vi "S8300E_BP_SoftRest_WIH.vi"() -> ()   [LabVIEW 2011]
panel:
  out "Prelog1":string
  out "prelog2":string
  out "log2":string
  out "FinalLog1":string
  out "LOG1":string
  out "FinalLog2":string
  out "Test CMD":T1(array[cluster])
  out "Init CMD":T2(array[cluster])
  out "VISA Handle Array":refnum<visa-resource-name>[](array[refnum])
  out "VISA6":refnum<visa-resource-name>
  out "VISA9":refnum<visa-resource-name>
  out "BEGIN TIME":u32
  out "進行狀況":string
  # "Error Code:BP-RST"
  # "S8300E BackPlane  SW Reset"
  # "2015-5-28"
  # "PC Com9 Baud  115200 -->S8300E MB\nPC COM6 Baud 115200 -->Test Board UART"
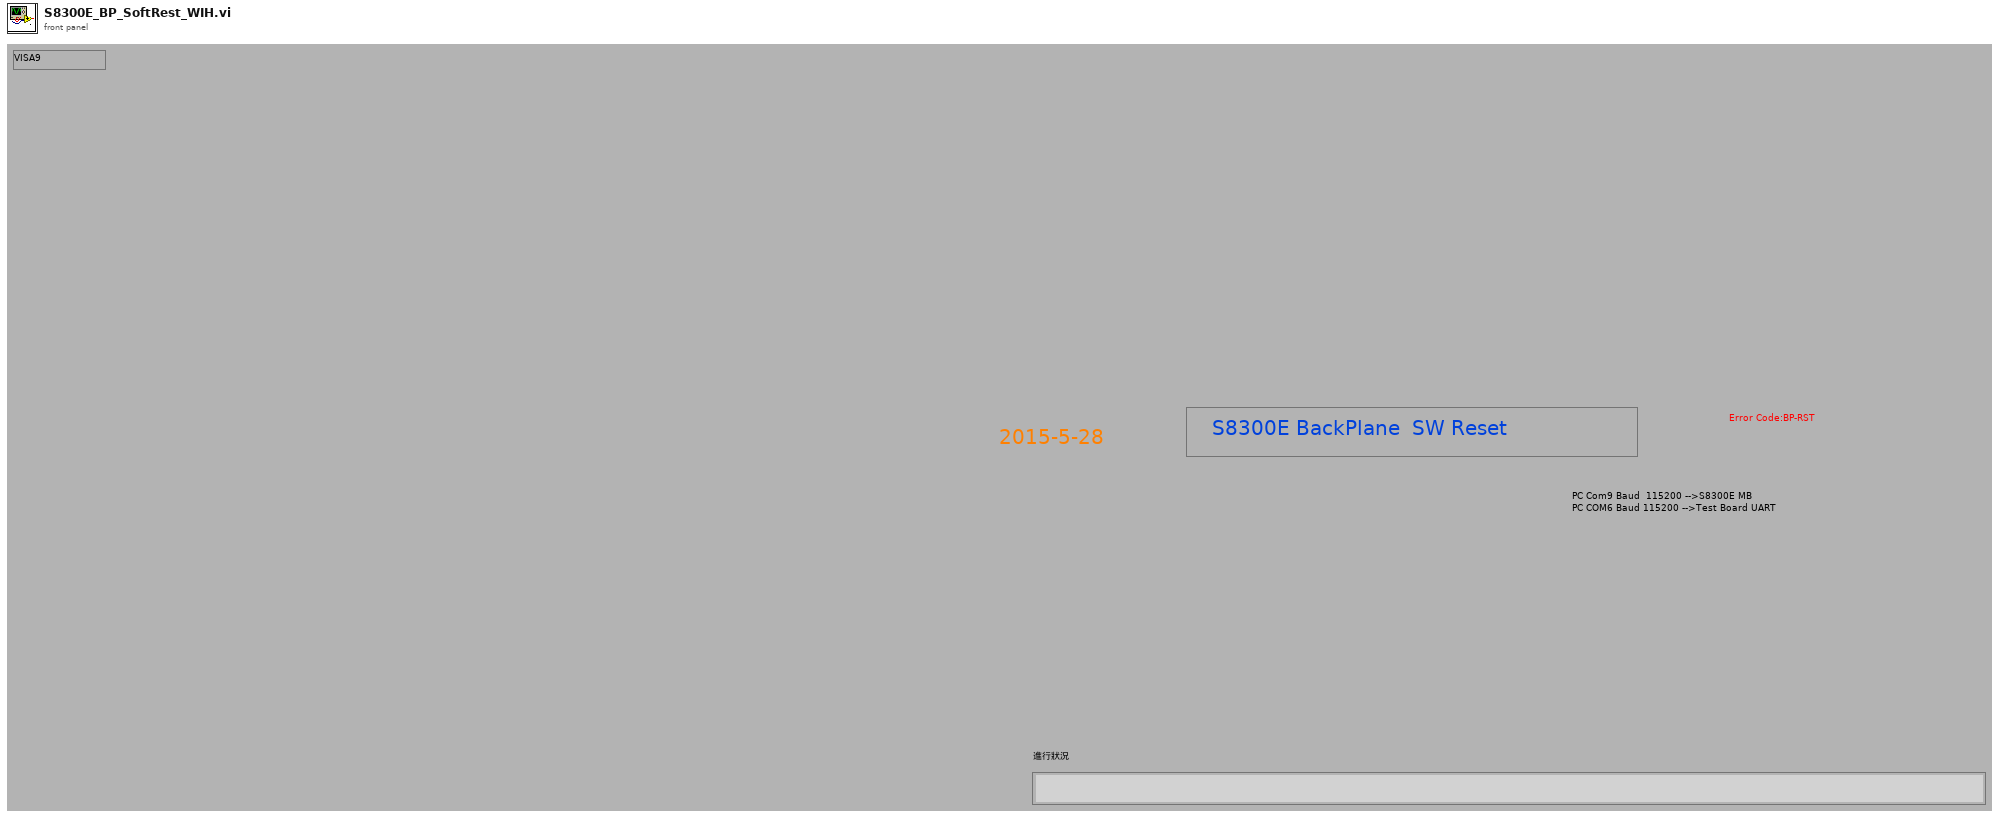
[diagram p1: front panel]
types:
  T1 = cluster{"VISA9":refnum<visa-resource-name>, "Find this String":string, "Find this String":string, "Find this String":string}[]
  T2 = cluster{"Find this String":string, "Find this String":string, "Find this String":string}[]
  T3 = cluster{string, "Find this String":string, "Find this String":string}
  T4 = cluster{"VISA6":refnum<visa-resource-name>, string, "Find this String":string, "Find this String":string}
  T5 = cluster{"VISA9":refnum<visa-resource-name>, string, "Find this String":string, "Find this String":string}
  T6 = cluster{string, "Find this String":string, "Find this String":string}[]
  T7 = cluster{"VISA6":refnum<visa-resource-name>, string, "Find this String":string, "Find this String":string}[]
  T8 = cluster{"Find this String":string, "Find this String":string, "Find this String":string}
  T9 = cluster{"VISA9":refnum<visa-resource-name>, "Find this String":string, "Find this String":string, "Find this String":string}
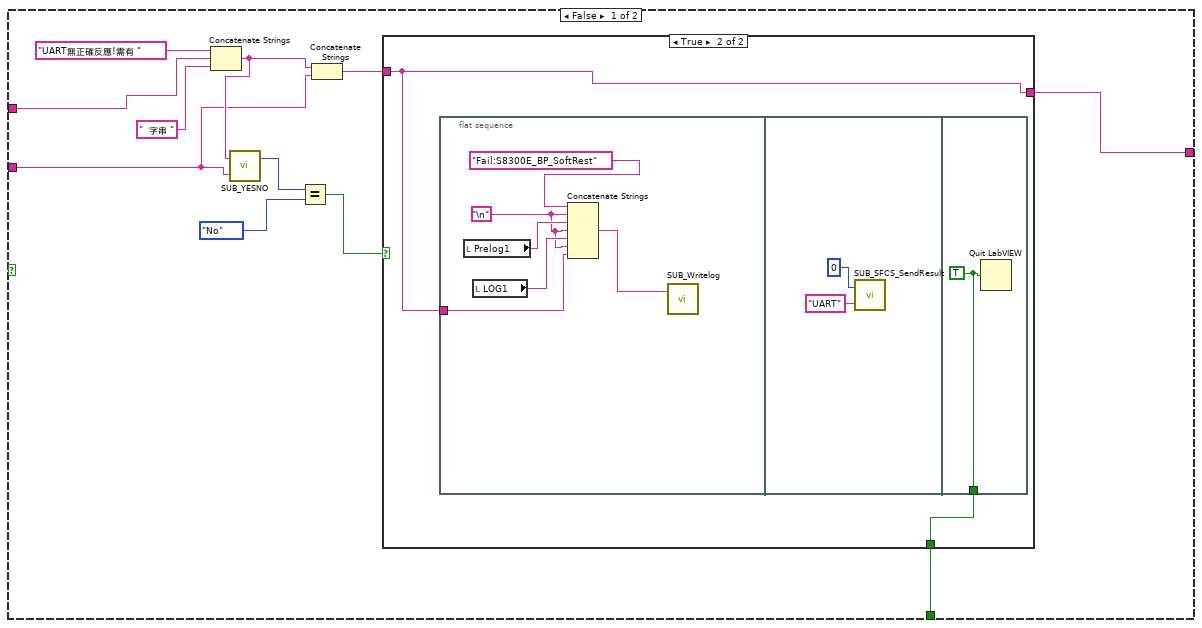
[diagram p3: hidden frame]
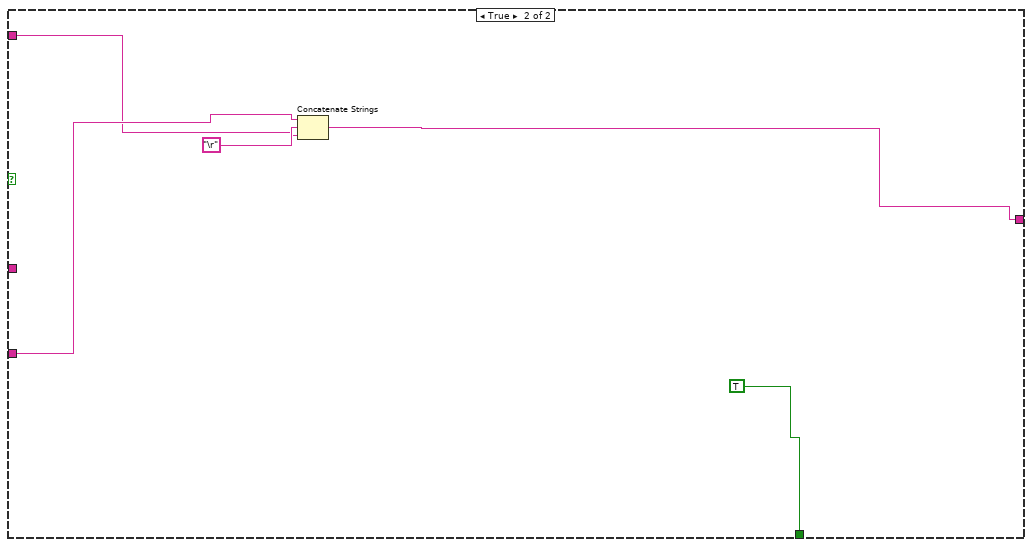
[diagram p6: hidden frame]
diagram:
  n1 = flat-sequence {
    tunnel: [w15] -> w4
    tunnel: w4 -> [w20]
    tunnel: [w20] -> w3
    tunnel: [w18] -> w2
    tunnel: w3 -> [w22]
    tunnel: w2 -> [w21]
    tunnel: [w122] -> w1
    tunnel: w1 -> [w123]
    frame #0 {
      n2 = Tick Count (ms)() -> (millisecond timer value=→"BEGIN TIME":u32)
    }
    frame #1 {
      n3 = Request Deallocation(TRUE ("flag")) -> ()
      n4 = property on="進行狀況" class="Str"("Blinking"=TRUE) -> ()  [unwired: 2 in, 2 out]
      "進行狀況" <- "進入測試準備中...." ("進行狀況")
    }
    frame #2 {
      n5 = call "SUB_SearchFile_inFolder.vi"("Search Filename in Folder"="S8300E_sfcs_misc.txt") -> ("File Existing True/Flase"=w9:bool)  [unwired: 1 in]
      n6 = case shown="False" w9 {
        frame False {
          n7 = flat-sequence {
            frame #0 {
              n8 = call "Display Message to User"() -> ()  [unwired: 10 in, 2 out]
            }
            frame #1 {
              n9 = call "SUB_Writelog.vi"("Pass/Fail"="Fail:S8300E_BP_SoftRest") -> ()  [unwired: 2 in]
            }
            frame #2 {
              n10 = Quit LabVIEW(quit? (T)=TRUE) -> ()
            }
          }
        }
        frame True {
        }
      }
    }
    frame #3 {
      n11 = call "SUB_COM1_CLOSE.vi"("VISA resource name"=refnum<visa-resource-name> "COM6") -> ()  [unwired: 3 in]
    }
    frame #4 {
      n12 = call "SUB_COM1_CLOSE.vi"("VISA resource name"=refnum<visa-resource-name> "COM9") -> ()  [unwired: 3 in]
    }
    frame #5 {
      n13 = call "SUB_COM_INIT.vi"("baud rate (9600)"=u32 115200, "VISA resource name"=refnum<visa-resource-name> "COM6") -> ("VISA resource name out"=w15:refnum<visa-resource-name>)  [unwired: 1 out]
      "VISA6" <- w15
    }
    frame #6 {
      n14 = call "SUB_COM9_INIT.vi"("baud rate"=u32 115200) -> ("VISA resource name out"=w18:refnum<visa-resource-name>)  [unwired: 1 in, 1 out]
    }
    frame #7 {
      n15 = Build Array(w22, w21) -> (→"VISA Handle Array":refnum<visa-resource-name>[])
      "VISA9" <- w21
    }
    frame #8 {
      w27 = "\r"
      w24 = "\r"
      w25 = "\r"
      n16 = local read "VISA6"() -> (w58:refnum<visa-resource-name>)
      n17 = Concatenate Strings("RT1" ("Find this String"), "\r") -> (w71:string)
      n18 = local read "VISA9"() -> (w31:refnum<visa-resource-name>)
      n19 = Concatenate Strings("RT0" ("Find this String"), "\r") -> (w62:string)
      n20 = local read "VISA6"() -> (w28:refnum<visa-resource-name>)
      n21 = Concatenate Strings("./bac.sh -r", w24, w24) -> (w61:string)
      n22 = Concatenate Strings("RT1" ("Find this String"), "\r") -> (w70:string)
      n23 = Concatenate Strings("./bac.sh -a", w27, w27) -> (w39:string)
      n24 = Concatenate Strings("RT1" ("Find this String"), "\r") -> (w48:string)
      n25 = Concatenate Strings("RT1" ("Find this String"), "\r") -> (w32:string)
      n26 = Concatenate Strings("./bac.sh -a", w25, w25) -> (w79:string)
      n27 = Concatenate Strings("./bac.sh -r", "\r") -> (w69:string)
      n28 = Bundle(w48, "Find this String"="RT1: Pass", "Find this String"="Checking COM6 Function...") -> (w74:T3)  [unwired: 1 in]
      n29 = Bundle("\r", "Find this String"="s8300e_func_test", "Find this String"="Checking COM9 Function") -> (w73:T3)  [unwired: 1 in]
      n30 = Bundle("VISA6"=w58, w70, "Find this String"="RT1: Pass", "Find this String"="G450 Output Signal Pattern RT1") -> (w56:T4)  [unwired: 1 in]
      n31 = Bundle("VISA9"=w31, w69, "Find this String"="PASSED=0x00", "Find this String"="Get Soft Reset (RST1) Event Indication") -> (w55:T5)  [unwired: 1 in]
      n32 = Bundle("VISA6"=w28, w32, "Find this String"="RT1: Pass", "Find this String"="G450 Output Signal Pattern RT1") -> (w29:T4)  [unwired: 1 in]
      n33 = Bundle("VISA6"=w58, w71, "Find this String"="RT1: Pass", "Find this String"="G450 Output Signal Pattern RT1") -> (w54:T4)  [unwired: 1 in]
      n34 = Bundle("VISA9"=w31, w79, "Find this String"="PASSED", "Find this String"="Set VLAN IP Address Interrupt Acknowledge") -> (w57:T5)  [unwired: 1 in]
      n35 = Bundle("VISA9"=w31, w61, "Find this String"="PASSED=0x01", "Find this String"="Get Soft Reset (RST1) Event Indication") -> (w52:T5)  [unwired: 1 in]
      n36 = Bundle("VISA9"=w31, w39, "Find this String"="PASSED", "Find this String"="Set VLAN IP Address Interrupt Acknowledge") -> (w30:T5)  [unwired: 1 in]
      n37 = Bundle("VISA6"=w58, w62, "Find this String"="RT0: Pass", "Find this String"="G450 Output Signal Pattern RT0") -> (w53:T4)  [unwired: 1 in]
      n38 = Build Array(w74, w73) -> (→"Init CMD":T6)
      n39 = Build Array(w57, w56, w55, w54, w53, w52, w30, w29) -> (→"Test CMD":T7)
    }
    frame #9 {
      n40 = while {
        shift-right: [w94] -> _
        shift-left: "" -> [w95]
        i -> [w99]
        stop <- w100 stop-if-true
        w93 = "Fail" ("Find this String")
        n41 = local read "VISA6"() -> (w88:refnum<visa-resource-name>)
        n42 = Greater Or Equal?(x=w99, y=3) -> (x >= y?=w97:bool)
        n43 = Tick Count (ms)() -> (millisecond timer value=w90:u32)
        n44 = call "SUB_WR_COM1_CbyCFindString_timeout.vi"("Begin time"=w90, "Find this String"=w93, "Timeout Seccond"=3.0, "cmd string"="\r", "duplicate VISA resource name 2"=w88) -> ("Output String"=w96:string, "Found String"=w92:bool)  [unwired: 2 out]
        n45 = Concatenate Strings(w95, w96) -> (w94:string)
        n46 = call "SUB_FindSpecificString.vi"("Find this String"=w93, "String data"=w94) -> ("Found"=w91:bool)  [unwired: 2 in, 1 out]
        n47 = Or(x=w92, y=w91) -> (x .or. y?=w89:bool)
        n48 = Or(x=w89, y=w97) -> (x .or. y?=w100:bool)
      }
    }
    frame #10 {
      n49 = local read "VISA6"() -> (w103:refnum<visa-resource-name>)
      n50 = call "SUB_COM_FLUSH_TXRX.vi"("VISA resource name"=w103) -> ()  [unwired: 2 in, 1 out]
    }
    frame #11 {
      n51 = while {
        shift-right: [w107] -> _
        shift-left: "" -> [w114]
        i -> [w108]
        stop <- w109 stop-if-true
        w106 = "RT1: Pass" ("Find this String")
        n52 = local read "VISA6"() -> (w118:refnum<visa-resource-name>)
        n53 = Concatenate Strings("RT1" ("string"), "\r") -> (w119:string)
        n54 = Greater Or Equal?(x=w108, y=3) -> (x >= y?=w112:bool)
        n55 = Tick Count (ms)() -> (millisecond timer value=w117:u32)
        n56 = call "SUB_WR_COM1_CbyCFindString_timeout.vi"("Begin time"=w117, "Find this String"=w106, "Timeout Seccond"=3.0, "cmd string"=w119, "duplicate VISA resource name 2"=w118) -> ("Output String"=w115:string, "Found String"=w105:bool)  [unwired: 2 out]
        n57 = Concatenate Strings(w114, w115) -> (w107:string)
        n58 = call "SUB_FindSpecificString.vi"("Find this String"=w106, "String data"=w107) -> ("Found"=w111:bool)  [unwired: 2 in, 1 out]
        n59 = Or(x=w105, y=w111) -> (x .or. y?=w110:bool)
        n60 = Or(x=w110, y=w112) -> (x .or. y?=w109:bool)
      }
    }
    frame #12 {
      n61 = Tick Count (ms)() -> (millisecond timer value=w122:u32)
    }
    frame #13 {
      n62 = while {
        shift-right: [w134] -> _
        shift-left: "" -> [w135]
        tunnel: w123 -> [w129]
        stop <- w132 stop-if-true
        n63 = local read "VISA9"() -> (w125:refnum<visa-resource-name>)
        n64 = call "SUB_COM1Wrt.vi"("VISA resource name"=w125, "write buffer"="\r") -> ("duplicate VISA resource name"=w138:refnum<visa-resource-name>)  [unwired: 1 in, 1 out]
        n65 = Tick Count (ms)() -> (millisecond timer value=w130:u32)
        n66 = Subtract(x=w130, y=w129) -> (x-y=w128:u32)
        n67 = Greater Or Equal?(x=w128, y=u32 5000) -> (x >= y?=w126:bool)
        n68 = call "SUB_ContinueCom1Read.vi"("Numeric"=1200, "duplicate VISA resource name 2"=w138) -> ("String"=w136:string)  [unwired: 1 in, 2 out]
        n69 = Concatenate Strings(w135, w136) -> (w134:string)
        n70 = call "SUB_FindSpecificString.vi"("Find this String"="S8300E", "String data"=w134) -> ("Found"=w131:bool)  [unwired: 2 in, 1 out]
        n71 = Or(x=w131, y=w126) -> (x .or. y?=w132:bool)
      }
    }
    frame #14 {
      n72 = local read "Init CMD"() -> (w143:T2)
      n73 = Array Size(array=w143) -> (size(s)=w142:i32)
      n74 = for {
        N: w142 -> [_]
        shift-right: [w147] -> w140
        shift-left: "" -> [w145]
        i -> [w150]
        n75 = local read "VISA Handle Array"() -> (w152:refnum<visa-resource-name>[])
        n76 = local read "Init CMD"() -> (w151:T2)
        n77 = Index Array(array=w152, index=w150) -> (element=w144:refnum<visa-resource-name>)
        n78 = Index Array(array=w151, index=w150) -> (element=w149:T8)
        n79 = while {
          tunnel: w149 -> [w167]
          shift-right: [w161] -> w146
          shift-left: "" -> [w160]
          tunnel: w144 -> [w154]
          stop <- w168 stop-if-true
          n80 = call "SUB_COM_FLUSH_TXRX.vi"("VISA resource name"=w154) -> ("VISA resource name out"=w153:refnum<visa-resource-name>)  [unwired: 2 in]
          n81 = Tick Count (ms)() -> (millisecond timer value=w163:u32)
          n82 = Unbundle(w167) -> ("Find this String"=w158:string, "Find this String"=w164:string, "Find this String"=w166:string)
          n83 = call "SUB_WR_COM1_CbyCFindString_timeout.vi"("Begin time"=w163, "Find this String"=w164, "Timeout Seccond"=5.0, "cmd string"=w158, "duplicate VISA resource name 2"=w153) -> ("Output String"=w155:string, "Found String"=w162:bool)  [unwired: 2 out]
          n84 = local write "進行狀況"(w166) -> ()
          n85 = Concatenate Strings(w158, "\n", w155) -> (w157:string)
          n86 = case shown="True" w162 {
            tunnel: [w176 TRUE] -> w168
            tunnel: w164 -> [w174 _]
            tunnel: w157 -> [w171 w192]
            tunnel: [w169 w192] -> w159
            frame False {
              n87 = Concatenate Strings("UART無正確反應!需有 " ("Status"), w174, "  字串 " ("Status")) -> (w172:string)
              n88 = call "SUB_YESNO.vi"("Debug View"=w171, "Status"=w172) -> ("yes/no"=w179:enum32{"No Selection", "Yes", "No", "None"})  [unwired: 1 in]
              n89 = Equal?(x=w179, y=enum32{"No Selection", "Yes", "No", "None"}."No") -> (x = y?=w177:bool)
              n90 = Concatenate Strings(w172, w171) -> (w170:string)
              n91 = case shown="True" w177 {
                tunnel: [_ w182] -> w176
                tunnel: w170 -> [w180 w181]
                tunnel: [w180 w181] -> w169
                frame False {
                }
                frame True {
                  n92 = flat-sequence {
                    tunnel: w181 -> [w183]
                    tunnel: [w191] -> w182
                    frame #0 {
                      w184 = "\n"
                      n93 = local read "Prelog1"() -> (w186:string)
                      n94 = local read "LOG1"() -> (w185:string)
                      n95 = Concatenate Strings("Fail:S8300E_BP_SoftRest" ("Pass/Fail"), w184, w186, w184, w185, w184, w183) -> (w187:string)
                      n96 = call "SUB_Writelog.vi"("Pass/Fail"=w187) -> ()  [unwired: 2 in]
                    }
                    frame #1 {
                      n97 = call "SUB_SFCS_SendResult.vi"("ErrorCode"="UART", "PASS_Fail (1/0)"=i8 0) -> ()  [unwired: 1 out]
                    }
                    frame #2 {
                      w191 = TRUE ("quit? (T)")
                      n98 = Quit LabVIEW(quit? (T)=w191) -> ()
                    }
                  }
                }
              }
            }
            frame True {
            }
          }
          n99 = Concatenate Strings(w160, w159) -> (w161:string)
          "LOG1" <- w161
        }
        n100 = Concatenate Strings(w145, w146) -> (w147:string)
        "Prelog1" <- w147
      }
      "FinalLog1" <- w140
    }
    frame #15 {
      n101 = local read "Test CMD"() -> (w197:T1)
      n102 = Array Size(array=w197) -> (size(s)=w196:i32)
      n103 = for {
        N: w196 -> [_]
        shift-right: [w201] -> w194
        shift-left: "" -> [w199]
        i -> [w202]
        n104 = while {
          tunnel: w202 -> [w217]
          shift-right: [w209] -> w200
          shift-left: "" -> [w207]
          stop <- w214 stop-if-true
          n105 = local read "Test CMD"() -> (w218:T1)
          n106 = Index Array(array=w218, index=w217) -> (element=w216:T9)
          n107 = Unbundle(w216) -> ("VISA9"=w204:refnum<visa-resource-name>, "Find this String"=w206:string, "Find this String"=w205:string, "Find this String"=w215:string)
          n108 = call "SUB_COM_FLUSH_TXRX.vi"("VISA resource name"=w204) -> ("VISA resource name out"=w203:refnum<visa-resource-name>)  [unwired: 2 in]
          n109 = local write "進行狀況"(w215) -> ()
          n110 = Tick Count (ms)() -> (millisecond timer value=w210:u32)
          n111 = call "SUB_WR_COM1_CbyCFindString_timeout.vi"("Begin time"=w210, "Find this String"=w205, "Timeout Seccond"=5.0, "cmd string"=w206, "duplicate VISA resource name 2"=w203) -> ("Output String"=w212:string, "Found String"=w211:bool)  [unwired: 2 out]
          n112 = case shown="False" w211 {
            tunnel: w212 -> [w222 w243]
            tunnel: [w224 TRUE] -> w214
            tunnel: [w220 w245] -> w208
            tunnel: w206 -> [_ w244]
            tunnel: w205 -> [w219 _]
            frame False {
              n113 = Concatenate Strings("系統需回" ("string"), w219) -> (w223:string)
              n114 = call "SUB_YESNO.vi"("Debug View"=w222, "Status"=w223) -> ("yes/no"=w228:enum32{"No Selection", "Yes", "No", "None"})  [unwired: 1 in]
              n115 = Equal?(x=w228, y=enum32{"No Selection", "Yes", "No", "None"}."No") -> (x = y?=w226:bool)
              n116 = Concatenate Strings(w223, w222) -> (w221:string)
              n117 = case shown="True" w226 {
                tunnel: [_ w231] -> w224
                tunnel: w221 -> [w229 w230]
                tunnel: [w229 w230] -> w220
                frame False {
                }
                frame True {
                  n118 = flat-sequence {
                    tunnel: w230 -> [w232]
                    tunnel: [w242] -> w231
                    frame #0 {
                      w233 = "\n"
                      n119 = local read "prelog2"() -> (w235:string)
                      n120 = local read "log2"() -> (w234:string)
                      n121 = Concatenate Strings("Fail:S8300E_BP_SoftRest" ("Pass/Fail"), w233, w235, w233, w234, w233, w232) -> (w236:string)
                      n122 = call "SUB_Writelog.vi"("Pass/Fail"=w236) -> ()  [unwired: 2 in]
                    }
                    frame #1 {
                      n123 = call "SUB_COM1_CLOSE.vi"("VISA resource name"=refnum<visa-resource-name> "COM6") -> ()  [unwired: 3 in]
                      n124 = call "SUB_SFCS_SendResult.vi"("ErrorCode"="BP-RST", "PASS_Fail (1/0)"=i8 0) -> ()  [unwired: 1 out]
                      n125 = call "SUB_COM1_CLOSE.vi"("VISA resource name"=refnum<visa-resource-name> "COM9") -> ()  [unwired: 3 in]
                    }
                    frame #2 {
                      w242 = TRUE ("quit? (T)")
                      n126 = Quit LabVIEW(quit? (T)=w242) -> ()
                    }
                  }
                }
              }
            }
            frame True {
              n127 = Concatenate Strings(w244, "\r", w243) -> (w245:string)
            }
          }
          n128 = Concatenate Strings(w207, w208) -> (w209:string)
          "log2" <- w209
        }
        n129 = Concatenate Strings(w199, w200) -> (w201:string)
        "prelog2" <- w201
      }
      "FinalLog2" <- w194
    }
    frame #16 {
      n130 = call "SUB_COM1_CLOSE.vi"("VISA resource name"=refnum<visa-resource-name> "COM6") -> ()  [unwired: 3 in]
    }
    frame #17 {
      w251 = "***Not Good ***" ("replace string (\"\")")
      w256 = "\n"
      n131 = local read "FinalLog1"() -> (w258:string)
      n132 = local read "FinalLog2"() -> (w257:string)
      n133 = local read "BEGIN TIME"() -> (w262:u32)
      n134 = Tick Count (ms)() -> (millisecond timer value=w261:u32)
      n135 = call "SUB_COM1_CLOSE.vi"("VISA resource name"=refnum<visa-resource-name> "COM9") -> ()  [unwired: 3 in]
      n136 = call "SUB_CAL_TESTTIME.vi"("Test Item name"="S8300E_BP_SoftRest", "Stop tick time"=w261, "Start tick time"=w262) -> ("Test Time output"=w255:string)  [unwired: 2 in]
      n137 = Concatenate Strings("Pass:S8300E_BP_SoftRest", w256, w258, w256, w257, w256, w255) -> (w250:string)
      n138 = call "SUB_SEARCH_REPLACE_STR.vi"("replace string (\"\")"=w251, "search string"="FAILED", "input string"=w250) -> ("result string"=w253:string)  [unwired: 2 in]
      n139 = call "SUB_SEARCH_REPLACE_STR.vi"("replace string (\"\")"=w251, "search string"="FAIL", "input string"=w253) -> ("result string"=w249:string)  [unwired: 2 in]
      n140 = call "SUB_Writelog.vi"("Pass/Fail"=w249) -> ()  [unwired: 2 in]
    }
    frame #18 {
      n141 = Quit LabVIEW(quit? (T)=TRUE ("stop? (T)")) -> ()
    }
  }
